vi "Write Send Image Msg.vi"(10 "UI.lvlib:Send Image Msg.lvclass":refnum<class "Send Image Msg.lvclass">, 11 "UI in":refnum<class "UI.lvclass">) -> (3 "UI out":refnum<class "UI.lvclass">)   [LabVIEW 2015, in "UI.lvlib" / "UI.lvclass"]
uses:
  UI.lvclass
  UI Messages/Send Image Msg/Send Image Msg.lvclass
  UI.lvclass/UI.ctl
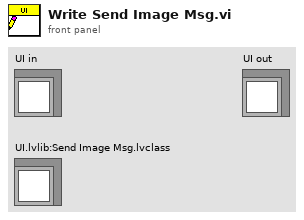
[diagram p1: front panel]
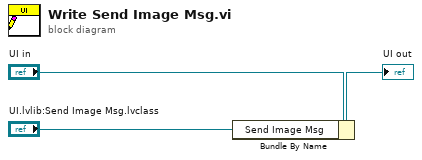
[diagram p0: block diagram]
diagram:
  n1 = Bundle By Name(cluster="UI in", "Send Image Msg"="UI.lvlib:Send Image Msg.lvclass") -> (→"UI out":refnum<class "UI.lvclass">)
